vi "initCSMs.vi"(7 "Enable building lvlibp?":bool, 8 "error in (no error)":errorcluster, 11 "TestCase in":refnum<class "testcase-CSMNonCSMCallerSupportAPI.lvclass">) -> (0 "error out":errorcluster, 3 "TestCase out":refnum<class "testcase-CSMNonCSMCallerSupportAPI.lvclass">)   [LabVIEW 2017, in "testcase-CSMNonCSMCallerSupportAPI.lvclass"]
uses:
  testcase-CSMNonCSMCallerSupportAPI.lvclass
  testcase-CSMNonCSMCallerSupportAPI.lvclass/testcase-CSMNonCSMCallerSupportAPI.ctl
  CSM/Normal-CSM.vi
  <vilib>/AppBuilder/AB_API_Simple/Build (path).vi
  CSM/Chain1.vi
  CSM/Chain2.vi
  CSM/Chain3.vi
  <vilib>/addons/_JKI Toolkits/VI Tester/TestCase.llb/TestCase.lvclass
  CSM/CSM-Testcase.lvlib
  src/user.lib/_NEVSTOP/Communicable State Machine(CSM)/Communicable State Machine.lvlib
  <vilib>/AppBuilder/AB_API_Simple/NI_App_Builder_API.lvlib
  C:/Program Files (x86)/National Instruments/LabVIEW 2017/vi.lib/addons/_JKI Toolkits/VI Tester/TestCase.llb/TestCase.lvclass
panel:
  out "Waited (ms)":u32
  out "CSMs Left":string[](array[string])
  out "Generated files":path[](array[path])
  out "CSMs":string[](array[string])
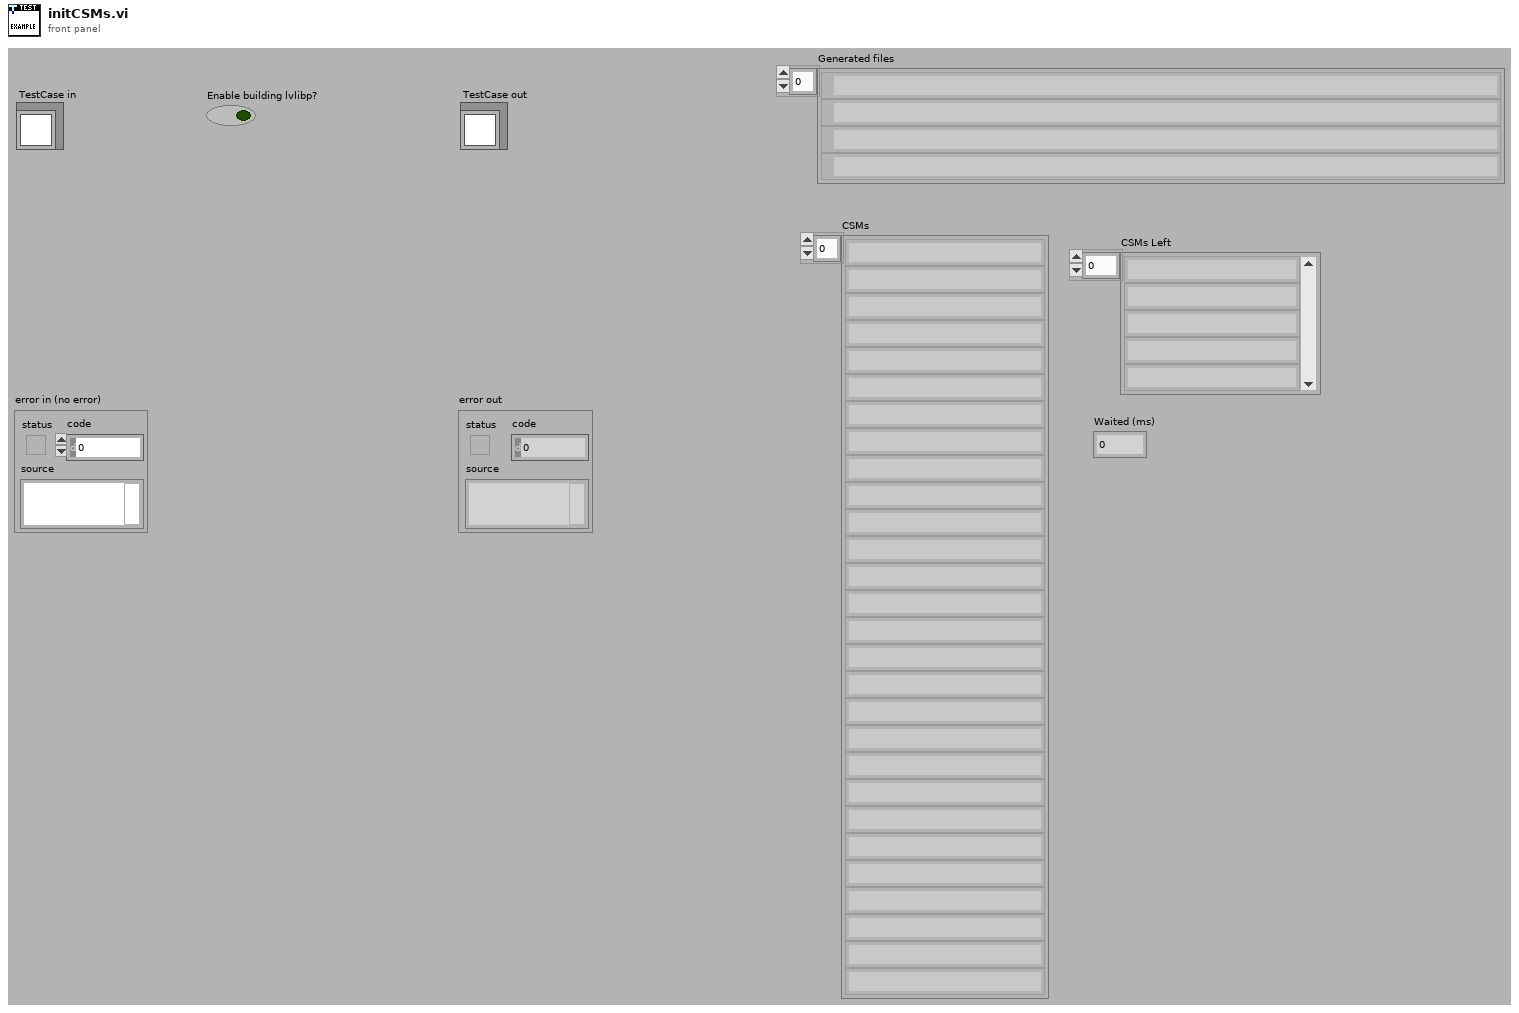
[diagram p1: front panel]
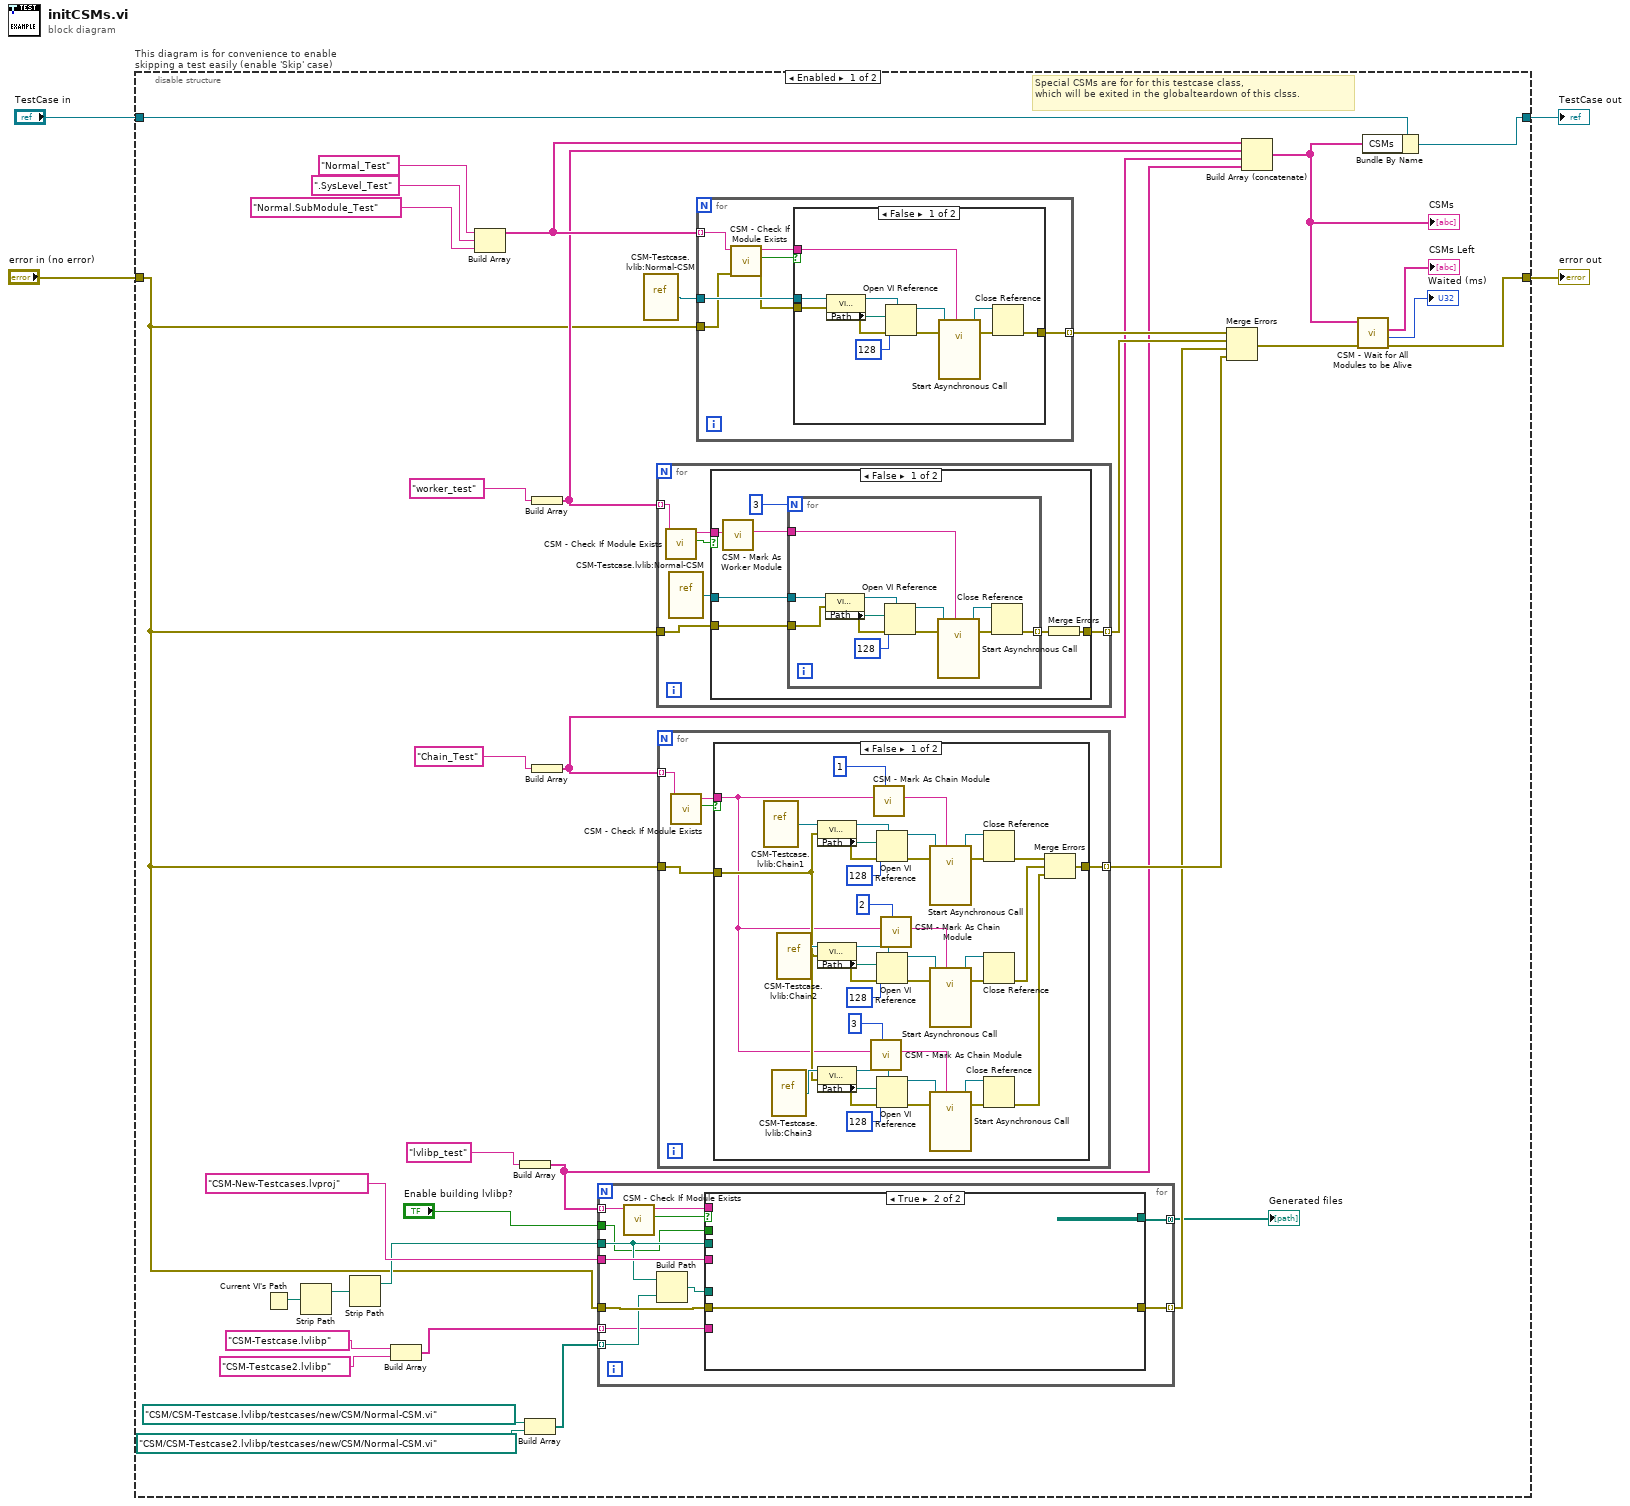
[diagram p0: block diagram]
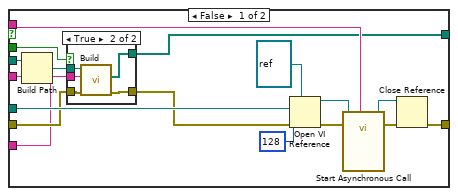
[diagram p2: hidden frame]
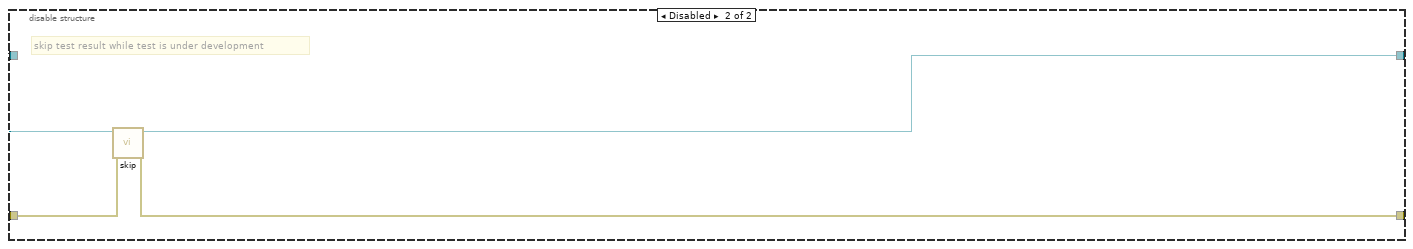
[diagram p7: hidden frame]
diagram:
  n1 = disable-structure "This diagram is for convenience to enable skipping a test easily (enable 'Skip' case)" shown="Enabled" {
    disable-tunnel: "TestCase in" -> [w7 w170]
    disable-tunnel: [w5 w168] -> w1
    disable-tunnel: [w8 w169] -> w3
    disable-tunnel: "error in (no error)" -> [w9 w167]
    frame Enabled {
      # "Special CSMs are for for this testcase class,\nwhich will be exited in the globalteardown of this clsss."
      n2 = Current VI's Path() -> (path=w35:path)
      n3 = Strip Path(path=w35) -> (stripped path=w36:path)  [unwired: 1 out]
      n4 = Strip Path(path=w36) -> (stripped path=w37:path)  [unwired: 1 out]
      n5 = Build Array("CSM-Testcase.lvlibp" ("Name of build specification (if empty: build all)"), "CSM-Testcase2.lvlibp" ("Name of build specification (if empty: build all)")) -> (w15:string[])
      n6 = Build Array("Normal_Test" ("Name (\"\" to Use UUID)"), ".SysLevel_Test" ("Name (\"\" to Use UUID)"), "Normal.SubModule_Test" ("Name (\"\" to Use UUID)")) -> (w31:string[])
      n7 = Build Array("lvlibp_test" ("Name (\"\" to Use UUID)")) -> (w21:string[])
      n8 = Build Array(path "CSM/CSM-Testcase.lvlibp/testcases/new/CSM/Normal-CSM.vi" ("vi path"), path "CSM/CSM-Testcase2.lvlibp/testcases/new/CSM/Normal-CSM.vi" ("vi path")) -> (w18:path[])
      n9 = Build Array("worker_test" ("Name (\"\" to Use UUID)")) -> (w25:string[])
      n10 = Build Array("Chain_Test" ("Name (\"\" to Use UUID)")) -> (w23:string[])
      n11 = for {
        tunnel: "CSM-New-Testcases.lvproj" ("name or relative path") -> [w49]
        tunnel: w37 -> [w44]
        tunnel: w21 -> [w46] mode=indexing
        tunnel: w18 -> [w45] mode=indexing
        tunnel: w15 -> [w42] mode=indexing
        tunnel: [w41] -> w14 mode=concatenating
        tunnel: "Enable building lvlibp?" -> [w40]
        tunnel: w9 -> [w50]
        tunnel: [w48] -> w34 mode=indexing
        n12 = call "CSM - Check If Module Exists.vi"("CSM Name"=w46) -> ("Exist?"=w51:bool, "CSM Name (Dup)"=w47:string)  [unwired: 8 in, 1 out]
        n13 = Build Path(base path=w44, name or relative path=w45) -> (appended path=w43:path)
        n14 = case shown="True" w51 {
          tunnel: [w68 w75] -> w48
          tunnel: w43 -> [w61 _]
          tunnel: w44 -> [w60 _]
          tunnel: w49 -> [w58 _]
          tunnel: w47 -> [w57 _]
          tunnel: w50 -> [w56 w75]
          tunnel: w42 -> [w54 _]
          tunnel: [w53 _] -> w41
          tunnel: w40 -> [w52 _]
          frame False {
            n15 = Build Path(base path=w60, name or relative path=w58) -> (appended path=w59:path)
            n16 = case shown="True" w52 {
              tunnel: w59 -> [_ w74]
              tunnel: w56 -> [w69 w73]
              tunnel: [w69 w72] -> w55
              tunnel: w54 -> [_ w71]
              tunnel: [_ w70] -> w53
              frame False {
              }
              frame True {
                n17 = call-poly <vilib>:"Build.vi"("error in (no error)"=w73, "Name of build specification (if empty: build all)"=w71, "Path to project"=w74) -> ("error out"=w72:errorcluster, "Generated files"=w70:path[])  [unwired: 7 in]
              }
            }
            n18 = Open VI Reference(type specifier VI Refnum (for type only)=refnum<vi> refnum ("reference out"), vi path=w61, options=128, error in (no error)=w55) -> (vi reference=w64:refnum<vi>, error out=w66:errorcluster)  [unwired: 2 in]
            n19 = call-by-ref "Start Asynchronous Call"(reference=w64, error in=w66, "Name (\"\" to Use UUID)"=w57) -> (reference out=w63:refnum<vi>, error out=w65:errorcluster)  [unwired: 11 in]
            n20 = Close Reference(reference=w63, error in (no error)=w65) -> (error out=w68:errorcluster)
          }
          frame True {
          }
        }
      }
      "Generated files" <- w14
      n21 = vi-ref "CSM-Testcase.lvlib:Normal-CSM.vi"() -> (w27:refnum<vi>)
      n22 = for {
        tunnel: w25 -> [w122] mode=indexing
        tunnel: w9 -> [w126]
        tunnel: [w123] -> w33 mode=indexing
        n23 = call "CSM - Check If Module Exists.vi"("CSM Name"=w122) -> ("Exist?"=w125:bool, "CSM Name (Dup)"=w124:string)  [unwired: 8 in, 1 out]
        n24 = vi-ref "CSM-Testcase.lvlib:Normal-CSM.vi"() -> (w121:refnum<vi>)
        n25 = case shown="False" w125 {
          tunnel: w121 -> [w133 _]
          tunnel: [w127 w146] -> w123
          tunnel: w126 -> [w129 w146]
          tunnel: w124 -> [w128 _]
          frame False {
            n26 = call "CSM - Mark As Worker Module.vi"("CSM Name"=w128) -> ("CSM Name (Marked As Worker)"=w130:string)  [unwired: 9 in]
            n27 = for {
              N: 3 -> [_]
              tunnel: w133 -> [w137]
              tunnel: w130 -> [w136]
              tunnel: [w135] -> w131 mode=indexing
              tunnel: w129 -> [w134]
              n28 = property class="VI (strict)"(reference=w137, error in=w134) -> (reference out=w143:refnum<vi>, error out=w141:errorcluster, "Path"=w140:path)
              n29 = Open VI Reference(type specifier VI Refnum (for type only)=w143, vi path=w140, options=128, error in (no error)=w141) -> (vi reference=w139:refnum<vi>, error out=w144:errorcluster)  [unwired: 2 in]
              n30 = call-by-ref "Start Asynchronous Call"(reference=w139, error in=w144, "Name (\"\" to Use UUID)"=w136) -> (reference out=w138:refnum<vi>, error out=w142:errorcluster)  [unwired: 11 in]
              n31 = Close Reference(reference=w138, error in (no error)=w142) -> (error out=w135:errorcluster)
            }
            n32 = Merge Errors(w131) -> (w127:errorcluster)
          }
          frame True {
          }
        }
      }
      n33 = for {
        tunnel: w23 -> [w76] mode=indexing
        tunnel: w9 -> [w80]
        tunnel: [w78] -> w39 mode=indexing
        n34 = call "CSM - Check If Module Exists.vi"("CSM Name"=w76) -> ("Exist?"=w79:bool, "CSM Name (Dup)"=w77:string)  [unwired: 8 in, 1 out]
        n35 = case shown="False" w79 {
          tunnel: [w83 w120] -> w78
          tunnel: w80 -> [w82 w120]
          tunnel: w77 -> [w81 _]
          frame False {
            n36 = vi-ref "CSM-Testcase.lvlib:Chain1.vi"() -> (w119:refnum<vi>)
            n37 = vi-ref "CSM-Testcase.lvlib:Chain3.vi"() -> (w101:refnum<vi>)
            n38 = vi-ref "CSM-Testcase.lvlib:Chain2.vi"() -> (w102:refnum<vi>)
            n39 = property class="VI (strict)"(reference=w119, error in=w82) -> (reference out=w116:refnum<vi>, error out=w114:errorcluster, "Path"=w113:path)
            n40 = property class="VI (strict)"(reference=w102, error in=w82) -> (reference out=w105:refnum<vi>, error out=w107:errorcluster, "Path"=w108:path)
            n41 = property class="VI (strict)"(reference=w101, error in=w82) -> (reference out=w98:refnum<vi>, error out=w96:errorcluster, "Path"=w95:path)
            n42 = call "CSM - Mark As Chain Module.vi"("Order"=3, "CSM Name"=w81) -> ("CSM Name (Marked As Chain)"=w89:string)  [unwired: 8 in]
            n43 = call "CSM - Mark As Chain Module.vi"("Order"=1, "CSM Name"=w81) -> ("CSM Name (Marked As Chain)"=w87:string)  [unwired: 8 in]
            n44 = Open VI Reference(type specifier VI Refnum (for type only)=w116, vi path=w113, options=128, error in (no error)=w114) -> (vi reference=w112:refnum<vi>, error out=w117:errorcluster)  [unwired: 2 in]
            n45 = Open VI Reference(type specifier VI Refnum (for type only)=w105, vi path=w108, options=128, error in (no error)=w107) -> (vi reference=w109:refnum<vi>, error out=w104:errorcluster)  [unwired: 2 in]
            n46 = Open VI Reference(type specifier VI Refnum (for type only)=w98, vi path=w95, options=128, error in (no error)=w96) -> (vi reference=w94:refnum<vi>, error out=w99:errorcluster)  [unwired: 2 in]
            n47 = call "CSM - Mark As Chain Module.vi"("Order"=2, "CSM Name"=w81) -> ("CSM Name (Marked As Chain)"=w88:string)  [unwired: 8 in]
            n48 = call-by-ref "Start Asynchronous Call"(reference=w112, error in=w117, "Name (\"\" to Use UUID)"=w87) -> (reference out=w111:refnum<vi>, error out=w115:errorcluster)  [unwired: 11 in]
            n49 = call-by-ref "Start Asynchronous Call"(reference=w109, error in=w104, "Name (\"\" to Use UUID)"=w88) -> (reference out=w110:refnum<vi>, error out=w106:errorcluster)  [unwired: 11 in]
            n50 = call-by-ref "Start Asynchronous Call"(reference=w94, error in=w99, "Name (\"\" to Use UUID)"=w89) -> (reference out=w93:refnum<vi>, error out=w97:errorcluster)  [unwired: 11 in]
            n51 = Close Reference(reference=w111, error in (no error)=w115) -> (error out=w92:errorcluster)
            n52 = Close Reference(reference=w110, error in (no error)=w106) -> (error out=w91:errorcluster)
            n53 = Close Reference(reference=w93, error in (no error)=w97) -> (error out=w90:errorcluster)
            n54 = Merge Errors(w92, w91, w90) -> (w83:errorcluster)
          }
          frame True {
          }
        }
      }
      n55 = for {
        tunnel: w27 -> [w153]
        tunnel: w31 -> [w149] mode=indexing
        tunnel: [w152] -> w32 mode=indexing
        tunnel: w9 -> [w151]
        n56 = call "CSM - Check If Module Exists.vi"("Error In"=w151, "CSM Name"=w149) -> ("error out"=w150:errorcluster, "Exist?"=w147:bool, "CSM Name (Dup)"=w148:string)  [unwired: 7 in]
        n57 = case shown="False" w147 {
          tunnel: w153 -> [w157 _]
          tunnel: [w156 w166] -> w152
          tunnel: w150 -> [w155 w166]
          tunnel: w148 -> [w154 _]
          frame False {
            n58 = property class="VI (strict)"(reference=w157, error in=w155) -> (reference out=w163:refnum<vi>, error out=w161:errorcluster, "Path"=w160:path)
            n59 = Open VI Reference(type specifier VI Refnum (for type only)=w163, vi path=w160, options=128, error in (no error)=w161) -> (vi reference=w159:refnum<vi>, error out=w164:errorcluster)  [unwired: 2 in]
            n60 = call-by-ref "Start Asynchronous Call"(reference=w159, error in=w164, "Name (\"\" to Use UUID)"=w154) -> (reference out=w158:refnum<vi>, error out=w162:errorcluster)  [unwired: 11 in]
            n61 = Close Reference(reference=w158, error in (no error)=w162) -> (error out=w156:errorcluster)
          }
          frame True {
          }
        }
      }
      n62 = Merge Errors(w32, w33, w34, w39) -> (w13:errorcluster)
      n63 = Build Array (concatenate)(w31, w25, w23, w21) -> (w6:string[])
      "CSMs" <- w6
      n64 = call "CSM - Wait for All Modules to be Alive.vi"("Error In"=w13, "CSM Names"=w6) -> ("error out"=w8:errorcluster, "Waited (ms)"=→"Waited (ms)":u32, "CSMs Left"=→"CSMs Left":string[])  [unwired: 7 in]
      n65 = Bundle By Name(cluster=w7, "CSMs"=w6) -> (w5:refnum<class "testcase-CSMNonCSMCallerSupportAPI.lvclass">)
    }
    frame Disabled {
      # "skip test result while test is under development"
      n66 = call <vilib>:"skip.vi"("error in (no error)"=w167, "TestCase in"=w170) -> ("error out"=w169:errorcluster, "TestCase out"=w168:refnum<class "testcase-CSMNonCSMCallerSupportAPI.lvclass">)  [unwired: 8 in]
    }
  }
  "error out" <- w3
  "TestCase out" <- w1
